vi "SeqMgr.Variables, Populate Variable Value Including Array Indices.vi"(8 "error in":errorcluster, 10 "String":string, 11 "Variables":variant) -> (0 "error out":errorcluster, 2 "String Out":string, 3 "Variables Out":variant)   [LabVIEW 2024, in "EQMF.lvlib" / "SeqMgr.lvlib"]
uses:
  SeqMgr.lvlib
panel:
  out "Indices Populated":string
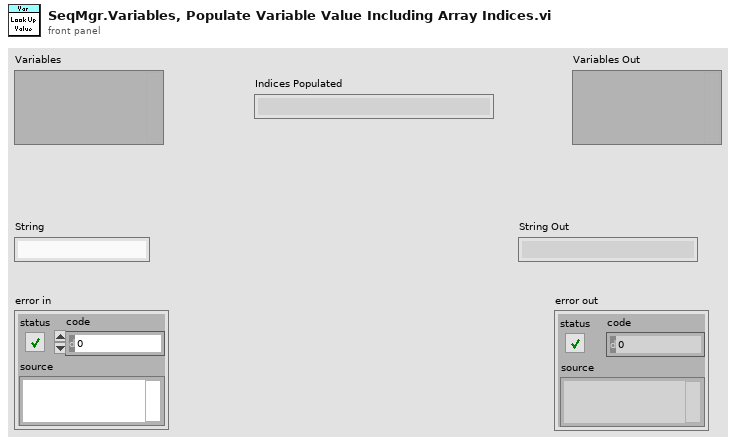
[diagram p1: front panel]
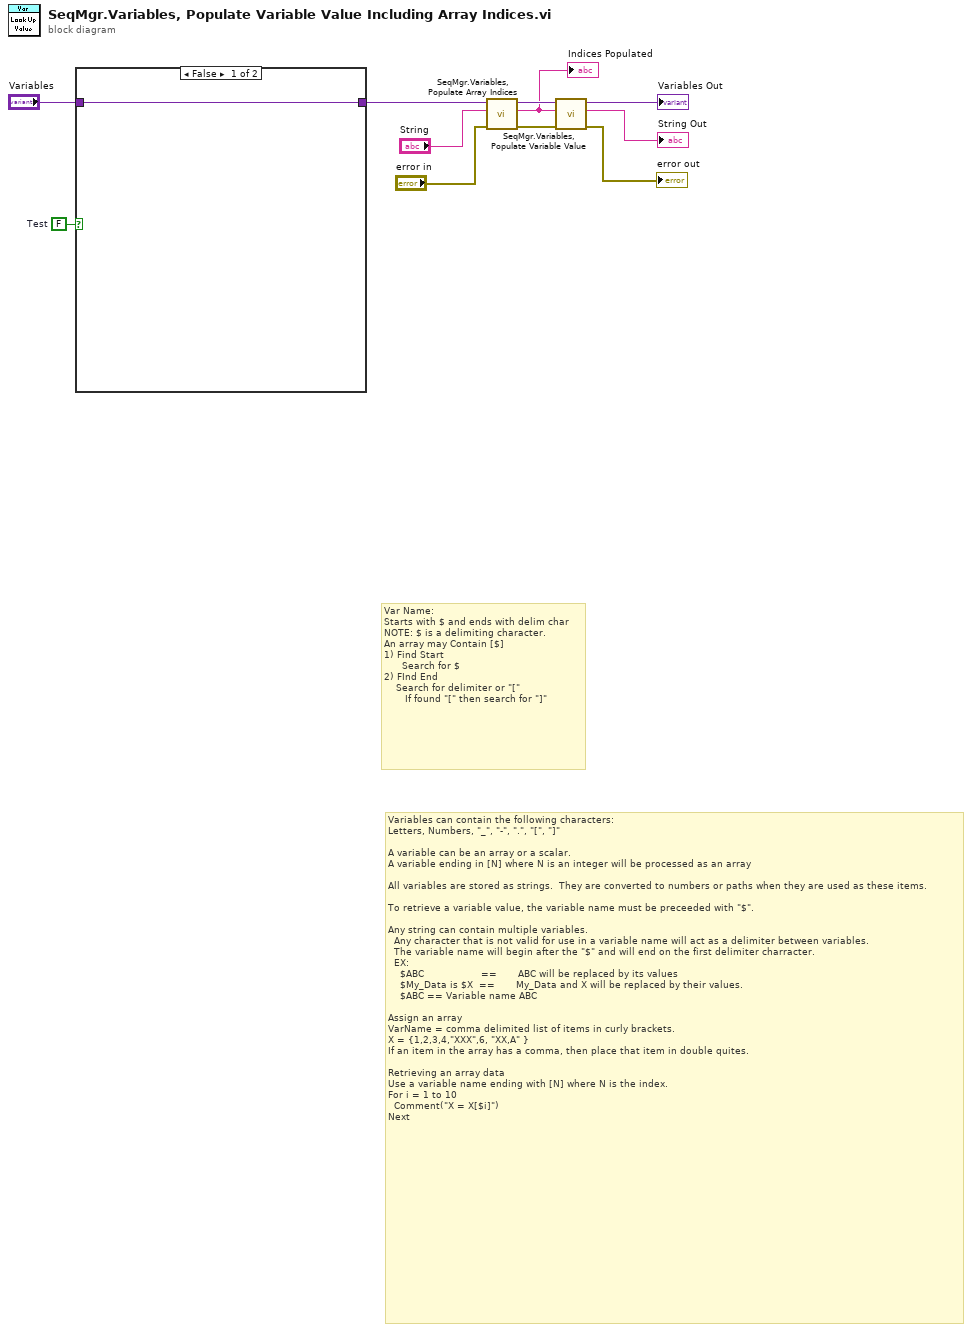
[diagram p0: block diagram]
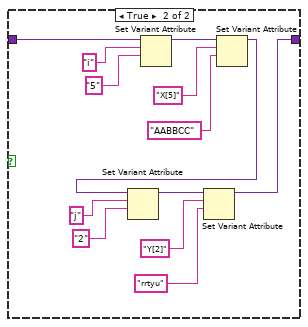
[diagram p2: hidden frame]
diagram:
  w1 = FALSE  # Test
  # "Var Name:\nStarts with $ and ends with delim char\nNOTE: $ is a delimiting character.\nAn array may Contain [$]\n1) Find Start\n      Search for $\n2) FInd End\n    Search for delimiter or \"[\"\n       If found \"[\" then search for \"]\""
  # "Variables can contain the following characters:\nLetters, Numbers, \"_\", \"-\", \".\", \"[\", \"]\"\n\nA variable can be an array or a scalar.\nA variable ending in [N] where N is an integer will be processed as an array\n\nAll variables are stored as strings.  They are converted to numbers or paths when they are used as these items.\n\nTo retrieve a variable value, the variable name must be preceeded with \"$\".\n\nAny string can contain multiple variables.\n  Any character that is not valid for use in a variable name will act as a delimiter between variables.\n  The variable name will begin after the \"$\" and will end on the first delimiter charracter.\n  EX:\n    $ABC                   ==       ABC will be replaced by its values\n    $My_Data is $X  ==       My_Data and X will be replaced by their values.\n    $ABC == Variable name ABC\n\nAssign an array\nVarName = comma delimited list of items in curly brackets.\nX = {1,2,3,4,\"XXX\",6, \"XX,A\" }\nIf an item in the array has a comma, then place that item in double quites.\n\nRetrieving an array data\nUse a variable name ending with [N] where N is the index.\nFor i = 1 to 10\n  Comment(\"X = X[$i]\")\nNext"
  n1 = case shown="False" w1 {
    tunnel: "Variables" -> [w12 w20]
    tunnel: [w12 w14] -> w2
    frame False {
    }
    frame True {
      n2 = Set Variant Attribute(Variant=w20, name="i", value="5") -> (Variant out=w23:variant)  [unwired: 1 in, 2 out]
      n3 = Set Variant Attribute(Variant=w23, name="X[5]", value="AABBCC") -> (Variant out=w13:variant)  [unwired: 1 in, 2 out]
      n4 = Set Variant Attribute(Variant=w13, name="j", value="2") -> (Variant out=w17:variant)  [unwired: 1 in, 2 out]
      n5 = Set Variant Attribute(Variant=w17, name="Y[2]", value="rrtyu") -> (Variant out=w14:variant)  [unwired: 1 in, 2 out]
    }
  }
  n6 = call "SeqMgr.Variables, Populate Array Indices.vi"("error in"="error in", "String"="String", "Variables"=w2) -> ("error out"=w8:errorcluster, "String Out"=w3:string, "Variables Out"=w9:variant)  [unwired: 6 in]
  "Indices Populated" <- w3
  n7 = call "SeqMgr.Variables, Populate Variable Value.vi"("error in"=w8, "String"=w3, "Variables"=w9) -> ("error out"=→"error out":errorcluster, "String Out"=→"String Out":string, "Variables Out"=→"Variables Out":variant)  [unwired: 6 in]
